vi "rqcBob Device Dialog.vi"(8 "error in":errorcluster, 10 "Compatible Devices List":string[][](array[string])) -> (0 "error out":errorcluster, 2 "Device Index":i32)   [LabVIEW 2019, in "rqcBob.lvclass"]
uses:
  rqcBob.lvclass
  <vilib>/Utility/error.llb/Error Cluster From Error Code.vi
  <vilib>/ErrorRing/Error Ring.xnode
panel:
  in  "Cancel Button":bool
  in  "OK Button":bool
  in  "Select device from list":i32(listbox)
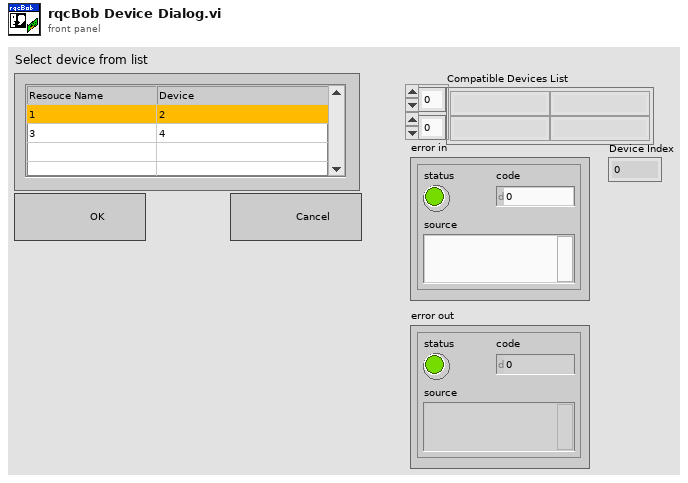
[diagram p1: front panel]
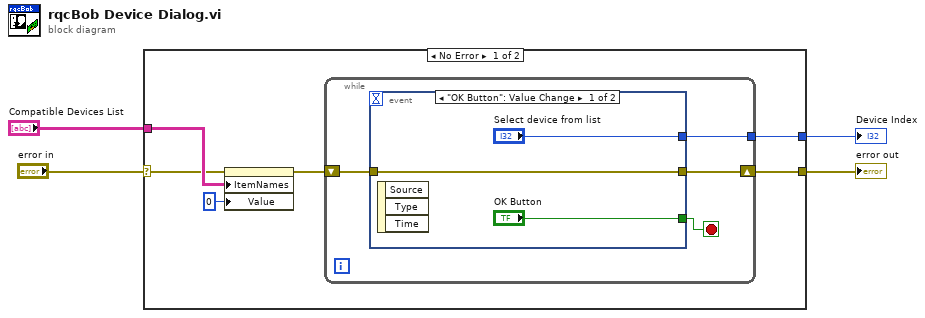
[diagram p0: block diagram]
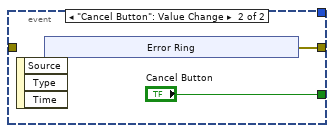
[diagram p2: hidden frame]
diagram:
  n1 = case shown="No Error" "error in" {
    selector: "error in" -> [w7 w24]
    tunnel: "Compatible Devices List" -> [w10 _]
    tunnel: [w6 w24] -> w2
    tunnel: [w5 _] -> w1
    frame No Error {
      n2 = property on="Select device from list" class="MCListbox (strict)"(error in=w7, "ItemNames"=w10, "Value"=0 ("Select device from list")) -> (error out=w8:errorcluster)  [unwired: 1 in, 1 out]
      n3 = while {
        tunnel: [w13] -> w5
        shift-right: [w12] -> w6
        shift-left: w8 -> [w11]
        stop <- w14 stop-if-true
        n4 = event shown="[0] \"OK Button\": Value Change" {
          selector: _ -> [_ _]
          dyn-events: _ -> [_ _]
          timeout: _ -> [_ _]
          tunnel: ["OK Button" "Cancel Button"] -> w14
          tunnel: ["Select device from list" _] -> w13
          tunnel: [w15 w18] -> w12
          tunnel: w11 -> [w15 _]
          event "OK Button": Value Change {
            n5 = event-data() -> ()  [unwired: 1 in, 3 out]
          }
          event "Cancel Button": Value Change {
            n6 = event-data() -> ()  [unwired: 1 in, 3 out]
            n7 = xnode "Error Ring"() -> ("error out"=w18:errorcluster)
          }
        }
      }
    }
    frame Error {
    }
  }
  "error out" <- w2
  "Device Index" <- w1
